vi "打地鼠.vi"() -> ()   [LabVIEW 2013]
uses:
  <vilib>/Utility/inputDevices.llb/mouseAcquire.vi
panel:
  out "win":bool
  out "目标分数":i32
  out "剩余时间":dbl
  out "数组":bool[][](array[boolean])
  out "分数":i32
  out "布尔":bool
  out "button 1":bool
  out "button info":T1 caption="按钮信息"
  out "axis info":T2 caption="坐标轴信息"
  in  "停止":bool
  # "左上角水平224 垂直152\n右下角水平822 垂直766\n场地的正方形区域是600*600大小，每个小正方形120*120\n坐标是（x,y）的老鼠，他的水平范围（224+120*x，224+120+20*x），\n垂直范围是（152+120*x,152+120+120*x）"
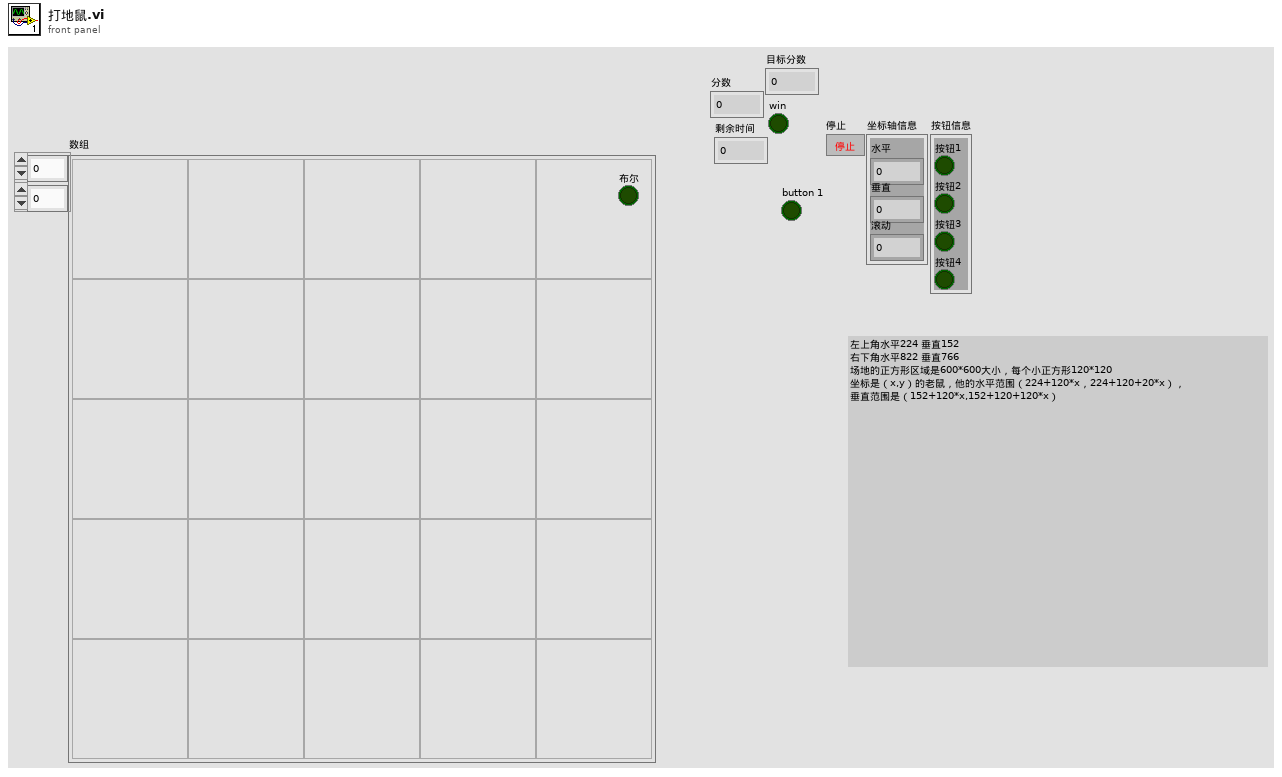
[diagram p1: front panel]
types:
  T1 = cluster{"button 1":bool, "button 2":bool, "button 3":bool, "button 4":bool}
  T2 = cluster{"Horizontal":i32, "Vertical":i32, "Scrolling":i32}
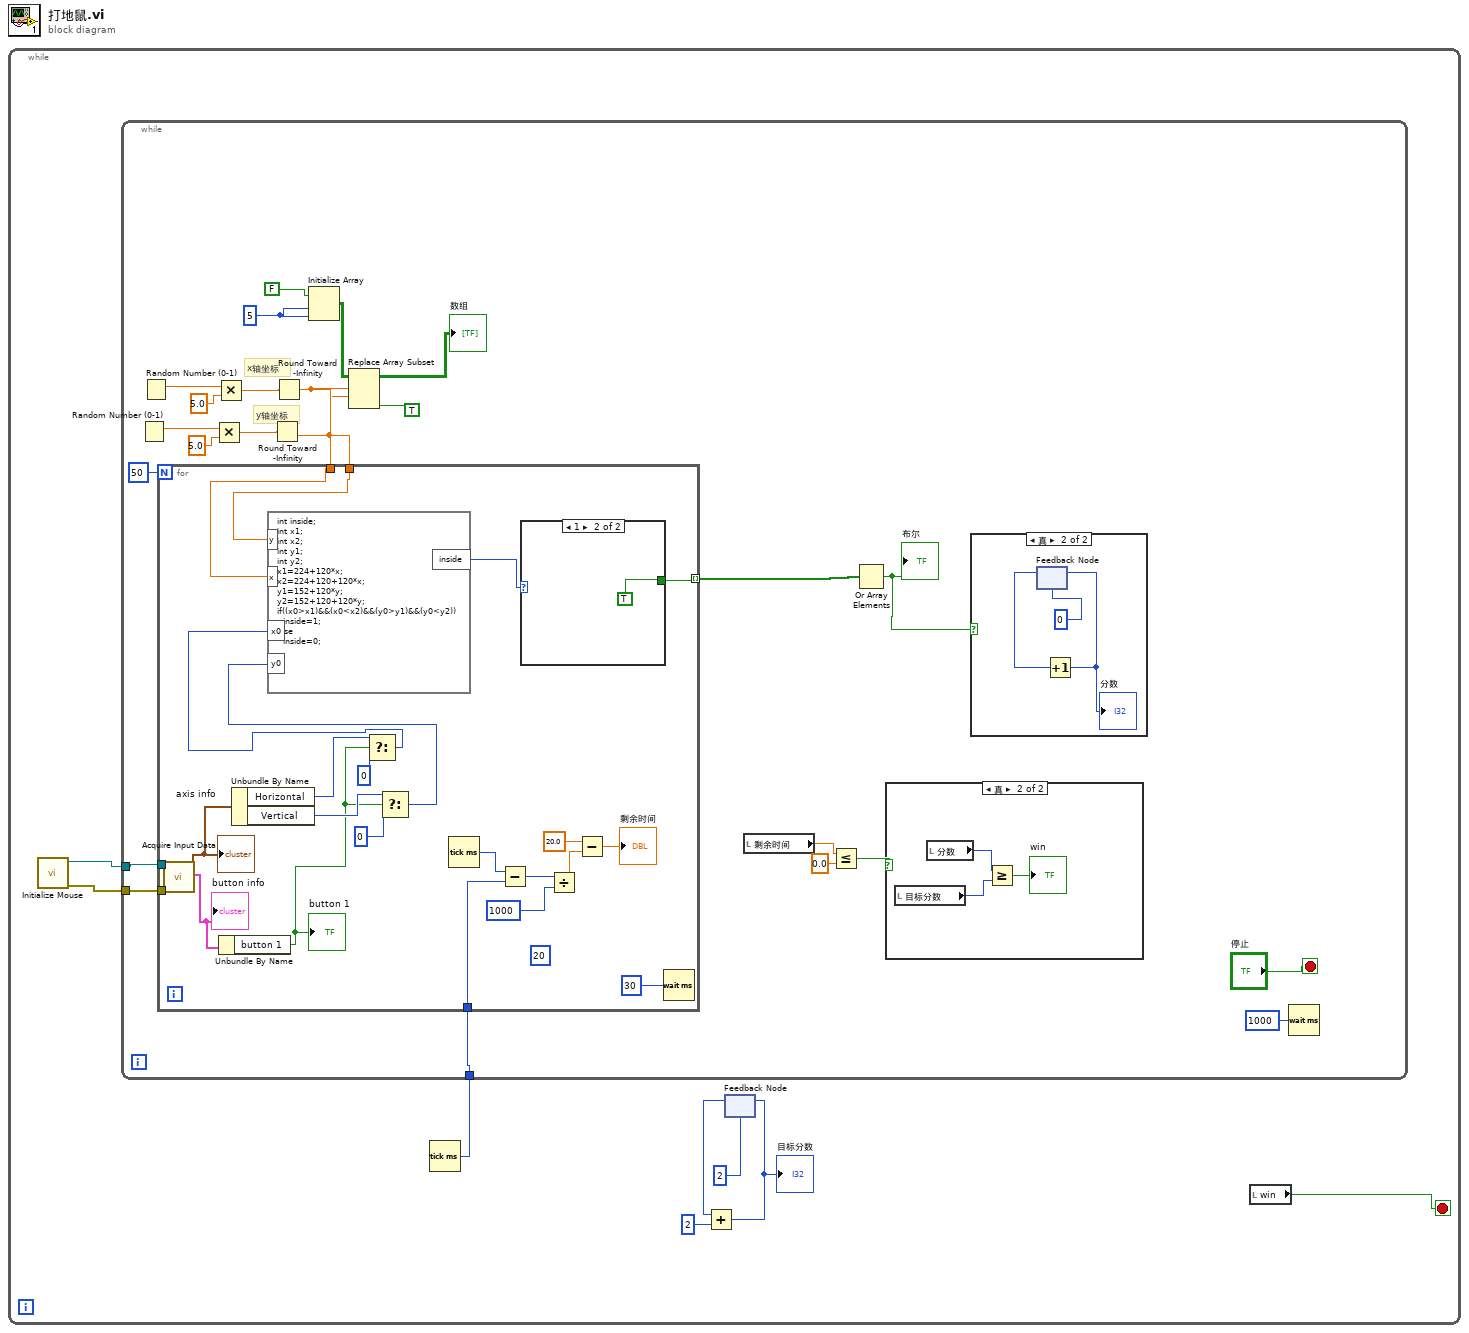
[diagram p0: block diagram]
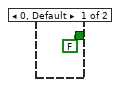
[diagram p4: hidden frame]
diagram:
  n1 = while {
    stop <- w5 stop-if-true
    n2 = call <vilib>:"Initialize Mouse.vi"() -> ("error out"=w7:errorcluster, "device ID"=w8:refnum<k1>)  [unwired: 10 in]
    n3 = Tick Count (ms)() -> (millisecond timer value=w6:u32)
    n4 = while {
      tunnel: w8 -> [w31]
      tunnel: w7 -> [w30]
      tunnel: w6 -> [w12]
      stop <- "停止" stop-if-true
      w15 = 5 ("维数大小")
      (unwired) u32 20 ("等待时间（毫秒）")
      # "y轴坐标"
      # "x轴坐标"
      n5 = Random Number (0-1)() -> (number: 0 to 1=w27:dbl)
      n6 = Random Number (0-1)() -> (number: 0 to 1=w24:dbl)
      n7 = Multiply(x=w27, y=5.0) -> (x*y=w26:dbl)
      n8 = Multiply(x=w24, y=5.0) -> (x*y=w25:dbl)
      n9 = Round Toward -Infinity(1:w26) -> (0:w21:dbl)
      n10 = Round Toward -Infinity(1:w25) -> (0:w22:dbl)
      n11 = for {
        N: 50 -> [_]
        tunnel: w31 -> [w61]
        tunnel: w30 -> [w60]
        tunnel: w22 -> [w50]
        tunnel: w21 -> [w51]
        tunnel: [w47] -> w18 mode=indexing
        tunnel: w12 -> [w44]
        n12 = call-poly <vilib>:"Acquire Input Data.vi"("device ID"=w61, "error in (no error)"=w60) -> ("axis info"=w59:T2, "button info"=w58:T1)  [unwired: 14 in, 2 out]
        "axis info" <- w59
        "button info" <- w58
        n13 = Unbundle By Name(w58) -> ("button 1"=w54:bool)
        "button 1" <- w54
        n14 = Unbundle By Name(w59) -> ("Horizontal"=w57:i32, "Vertical"=w55:i32)
        n15 = Select(t=w57, s=w54, f=0) -> (s? t:f=w48:i32)
        n16 = Select(t=w55, s=w54, f=0) -> (s? t:f=w49:i32)
        n17 = formula code="int inside;\nint x1;\nint x2;\nint y1;\nint y2;\nx1=224+120*x;\nx2=224+120+120*x;\ny1=152+120*y;\ny2=152+120+120*y;\nif((x0>x1)&&(x0<x2)&&(y0>y1)&&(y0<y2))\n  inside=1;\nelse\n  inside=0;"("y"=w51, "x"=w50, "x0"=w48, "y0"=w49) -> ("inside"=w46:i32)
        n18 = Tick Count (ms)() -> (millisecond timer value=w45:u32)
        n19 = Subtract(x=w45, y=w44) -> (x-y=w42:u32)
        n20 = case shown="1" w46 {
          tunnel: [FALSE TRUE] -> w47
          frame 0, Default {
          }
          frame 1 {
          }
        }
        n21 = Divide(x=w42, y=u32 1000) -> (x/y=w41:dbl)
        n22 = Subtract(x=20.0, y=w41) -> (x-y=→"剩余时间":dbl)
        n23 = Wait (ms)(milliseconds to wait=u32 30 ("等待时间（毫秒）")) -> ()  [unwired: 1 out]
      }
      n24 = Initialize Array(FALSE, w15, w15) -> (w14:bool[][])
      n25 = Replace Array Subset(array=w14, new element=TRUE, index (row)=w22, index (col)=w21) -> (→"数组":bool[][])
      n26 = local read "剩余时间"() -> (w11:dbl)
      n27 = Less Or Equal?(x=w11, y=0.0) -> (x <= y?=w9:bool)
      n28 = Or Array Elements(Boolean array=w18) -> (logical OR=w17:bool)
      "布尔" <- w17
      n29 = case shown="真" w9 {
        frame False {
        }
        frame True {
          n30 = local read "目标分数"() -> (w34:i32)
          n31 = local read "分数"() -> (w35:i32)
          n32 = Greater Or Equal?(x=w35, y=w34) -> (x >= y?=→"win":bool)
        }
      }
      n33 = case shown="真" w17 {
        frame False {
        }
        frame True {
          n34 = feedback #1(0) -> (w37:i32)
          n35 = Increment(x=w37) -> (x+1=w36:i32)
          "分数" <- w36
          n36 = feedback-in #1(w36) -> ()
        }
      }
      n37 = Wait (ms)(milliseconds to wait=u32 1000 ("等待时间（毫秒）")) -> ()  [unwired: 1 out]
    }
    n38 = feedback #2(2) -> (w2:i32)
    n39 = Add(x=w2, y=2) -> (x+y=w4:i32)
    "目标分数" <- w4
    n40 = feedback-in #2(w4) -> ()
    n41 = local read "win"() -> (w5:bool)
  }
